vi "Create Session.vi"(8 "error in (no error)":errorcluster, 11 "Session Id":u64) -> (0 "error out":errorcluster, 1 "Run Time Configuration":string, 2 "Edit Time Configuration":string, 3 "Session out":refnum<class "Plugin Session.lvclass">, 4 "Panel Size":T1)   [LabVIEW 2023, in "InstrumentStudio Plugin SDK.lvlib" / "Plugin Session.lvclass"]
doc: "Call this VI with the Session Id as the first SDK call at the beginning of your plugin VI. This VI sets up the events and other data needed for the plugin panel and framework to communicate. If you need to know the panel size for your plugin panel to adjust its front panel, this VI will return the size. Some plugin panels support both large and small panel sizes and need to adjust the visuals on their front panel to better fit into that panel size. LabVIEW plugin panels are uniquely identified by the Plugin Session which is set by the framework when the plugin is run. Plugins must have a control named 'Session Id' which is a U64 numeric control on their plugin VI front panel so the framework can correctly set it. This 'Session Id' is then passed to Create Session.vi to begin the plugin session. This control can be placed on the user's VI by right-clicking on the input of the Create Session.vi and choosing 'Create Control'.\nThe Plugin Session returned is then used to call other SDK VIs during execution of the plugin VI to get or set properties of the plugin panel or to notify the framework of various events."
uses:
  Plugin Session.lvclass
  Panel Size.ctl
  Plugin Events.ctl
  Event Registration Refnum.ctl
  Plugin Session.lvclass/Plugin Session.ctl
  Read Edit Time Configuration.vi
  Read Run Time Configuration.vi
  InstrumentStudio Plugin SDK.lvlib
  NationalInstruments.VIHost.Interop.dll
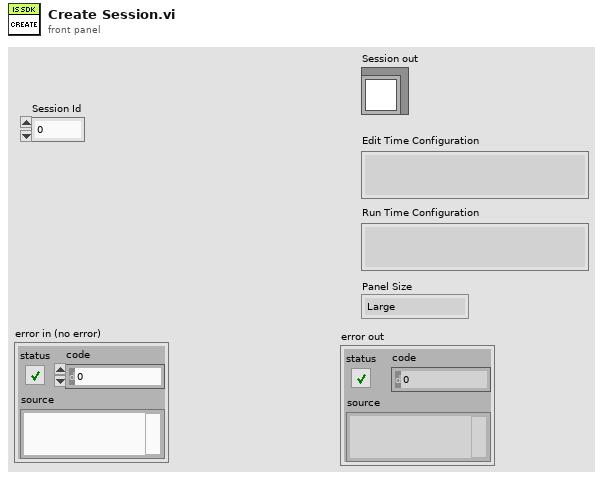
[diagram p1: front panel]
types:
  T1 = typedef "InstrumentStudio Plugin SDK.lvlib/Panel Size.ctl" = enum32{"Large", "Small"}
  T2 = typedef "InstrumentStudio Plugin SDK.lvlib/Plugin Events.ctl" = cluster{"Shutdown":refnum<user-event>, "Project Saved":refnum<user-event>, "Stop All Outputs":refnum<user-event>}
  T3 = typedef "InstrumentStudio Plugin SDK.lvlib/Event Registration Refnum.ctl" = refnum<event-registration>
  T4 = cluster{"Session Id":u64, "Plugin Events":T2, "Event Refnum":T3}
  T5 = cluster{"Project Path":path, "Completion Id":i64}
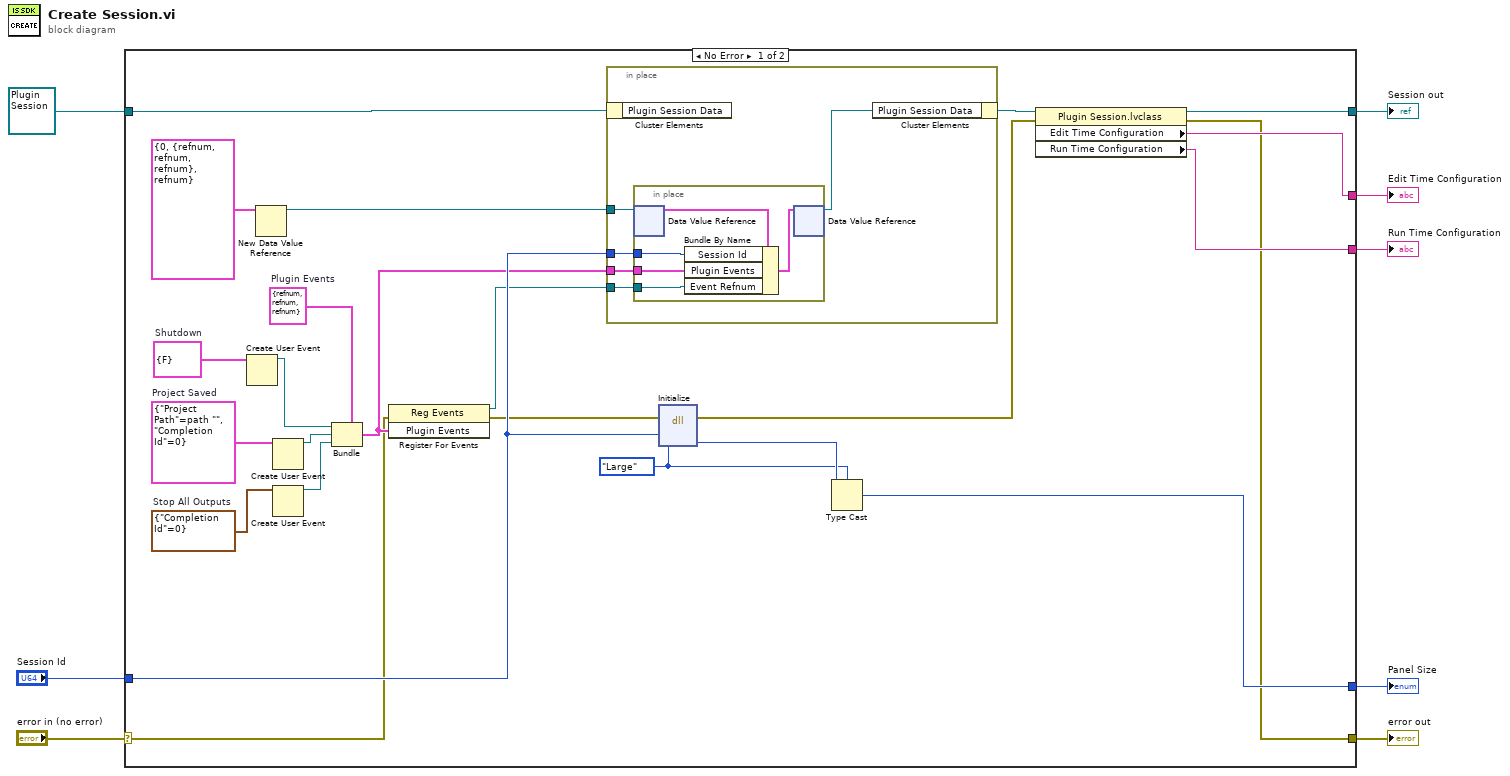
[diagram p0: block diagram]
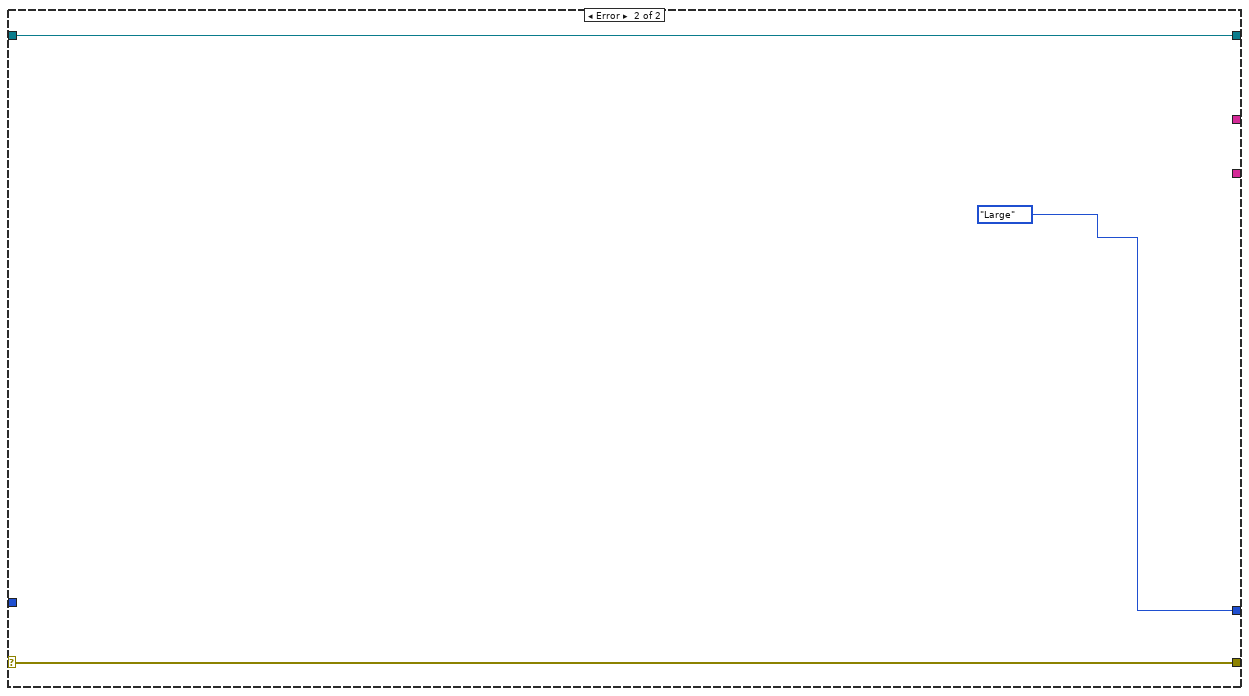
[diagram p2: hidden frame]
diagram:
  n1 = case shown="No Error" "error in (no error)" {
    selector: "error in (no error)" -> [w20 w44]
    tunnel: [w14 w44] -> w8
    tunnel: [w30 Panel_Size."Large" ("Panel Size")] -> w7
    tunnel: "Session Id" -> [w25 _]
    tunnel: refnum<class "Plugin Session.lvclass"> refnum ("PluginSDK:PluginSession.lvclass") -> [w22 w43]
    tunnel: [w15 w43] -> w3
    tunnel: [w18 _] -> w2
    tunnel: [w16 _] -> w1
    frame No Error {
      w12 = cluster{"Unused":bool} {"Unused"=FALSE}  # Shutdown
      w26 = T2 {"Shutdown"=refnum, "Project Saved"=refnum, "Stop All Outputs"=refnum}  # Plugin Events
      w28 = T5 {"Project Path"=path "", "Completion Id"=0}  # Project Saved
      w29 = cluster{"Completion Id":i64} {"Completion Id"=0}  # Stop All Outputs
      w31 = Panel_Size."Large" ("Panel Size")
      n2 = Create User Event(user event datatype=w12) -> (user event=w11:refnum<user-event>)  [unwired: 1 in, 1 out]
      n3 = New Data Value Reference(data value=T4 {"Session Id"=0, "Plugin Events"={"Shutdown"=refnum, "Project Saved"=refnum, "Stop All Outputs"=refnum}, "Event Refnum"=refnum} ("Cluster of class private data")) -> (data value reference=w27:refnum<data-value>)  [unwired: 1 in, 1 out]
      n4 = Create User Event(user event datatype=w28) -> (user event=w10:refnum<user-event>)  [unwired: 1 in, 1 out]
      n5 = Create User Event(user event datatype=w29) -> (user event=w9:refnum<user-event>)  [unwired: 1 in, 1 out]
      n6 = Bundle(cluster=w26, "Shutdown"=w11, "Project Saved"=w10, "Stop All Outputs"=w9) -> (w24:T2)
      n7 = register-events(error in=w20, w24) -> (reference out=w23:refnum<event-registration>, error out=w21:errorcluster)  [unwired: 1 in]
      n8 = in-place {
        in-place-border: w27 -> [w37]
        in-place-border: w25 -> [w36]
        in-place-border: w24 -> [w35]
        in-place-border: w23 -> [w34]
        n9 = in-place-cluster #1(w22) -> ()  [unwired: 1 out]
        n10 = in-place {
          in-place-border: w36 -> [w41]
          in-place-border: w35 -> [w40]
          in-place-border: w34 -> [w39]
          n11 = in-place-dvr #2(w37) -> (w42:T4)  [unwired: 1 out]
          n12 = Bundle By Name(cluster=w42, "Session Id"=w41, "Plugin Events"=w40, "Event Refnum"=w39) -> (w38:T4)
          n13 = in-place-dvr #2(w38) -> (w33:refnum<data-value>)  [unwired: 1 out]
        }
        n14 = in-place-cluster #1("Plugin Session Data"=w33) -> (w17:refnum<class "Plugin Session.lvclass">)
      }
      n15 = dll-call lib="C:/Users/nmurphy/Downloads/InstrumentStudio_LabVIEW_Plugins/LabVIEW/ExampleProject/PluginSDK/NationalInstruments.VIHost.Interop.dll" fn="Initialize"(error in=w21, "hostId"=w25, "panelSize"=w31) -> (error out=w13:errorcluster, "panelSize"=w32:u32)  [unwired: 4 in, 1 out]
      n16 = Type Cast(type=w31, x=w32) -> (*(type *) &x=w30:T1)
      n17 = property class="Plugin Session.lvclass"(reference=w17, error in=w13) -> (reference out=w15:refnum<class "Plugin Session.lvclass">, error out=w14:errorcluster, "Edit Time Configuration"=w18:string, "Run Time Configuration"=w16:string)
    }
    frame Error {
    }
  }
  "error out" <- w8
  "Panel Size" <- w7
  "Session out" <- w3
  "Edit Time Configuration" <- w2
  "Run Time Configuration" <- w1
